vi "CRYReplace Stimulus Curve Name.vi"(7 "Setup in":T1={"No.VI"=0, "Category"="", "StepName"="", "Seq setup flattened"="", "Comment"="", "Steps config."=[], "Jump config"=[], "Start"=0.0, "Increment"=0.0, "Name"="Pa", "Unit"="Pa", "Y data"=1, "Y prefix"="", "Y dB ref"=1.0, "Y unit"="", "Repeat State Array"=[]} {"Repeat State Array"."Start" format="%#_5g"; "Y dB ref" format="%.1f"; "Y data" items=["dB", "Lin"]; "Start" format="%#_5g"}, 8 "Hardware Setup In":string, 9 "Step Setup In":string, 11 "Type In":string) -> (3 "Inserted Names Out":string[](array[string]))   [LabVIEW 2013]
uses:
  Typedef Control/CRYData Variant Array.ctl
  Typedef Control/CRYWaveform Cluster.ctl
  Typedef Control/CRYStep.ctl
  Typedef Control/CRYData Cluster.ctl
panel:
  in  "Wave out":T2[](array[typedef]) {"Y dB ref" format="%.1f"; "Y axis" items=["Log", "Lin"]; "Y data" items=["dB", "Lin"]; "X data" items=["dB", "Lin"]}
  in  "Data In":T3
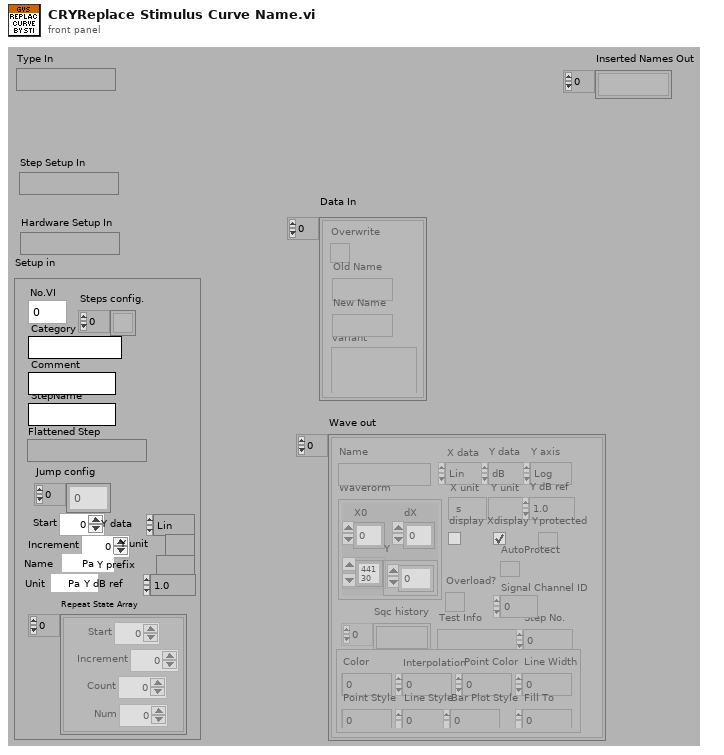
[diagram p1: front panel]
types:
  T1 = typedef "CRYStep.ctl" = cluster{"No.VI":i32, "Category":string, "StepName":string, "Seq setup flattened":string, "Comment":string, "Steps config.":bool[], "Jump config":i32[], "Start":dbl, "Increment":dbl, "Name":string, "Unit":string, "Y data":u16, "Y prefix":string, "Y dB ref":dbl, "Y unit":string, "Repeat State Array":cluster{"Start":dbl, "Increment":dbl, "Count":i32, "Num":i32}[]}
  T2 = typedef "CRYWaveform Cluster.ctl" = cluster{"Waveform":cluster{"X0":dbl, "dX":dbl, "Y":sgl[]}, "X data":u16, "Y data":u16, "Y axis":u16, "X unit":string, "Y unit":string, "Y dB ref":dbl, "display Y":bool, "display X":bool, "Overload?":bool, "Test Info":string, "Step No.":i32, "Name":string, "protected":bool, "Sqc history":string[], "Signal Channel ID":i32, "Plot Settings":cluster{"Color":u32, "Interpolation":u8, "Point Style":u8, "Line Style":u8, "Point Color":u32, "Line Width":u8, "Bar Plot Style":u8, "Fill To":i16}, "AutoProtect":bool}
  T3 = typedef "CRYData Variant Array.ctl" = cluster{"variant":variant, "Overwrite":bool, "Old Name":string, "New Name":string}[]
  T4 = typedef "CRYData Cluster.ctl" = cluster{"Name":string, "Curve":cluster{"x":dbl, "y":dbl, "z":dbl}[], "X data":u16, "Y data":u16, "Z data":u16, "X axis":u16, "Y axis":u16, "Z axis":u16, "X unit":string, "Y unit":string, "Z unit":string, "X dB ref":dbl, "Y dB ref":dbl, "Z dB ref":dbl, "single val":bool, "protected":bool, "display X":bool, "display Y":bool, "display Z":bool, "Test Info":string, "Step No.":i32, "Plot Settings":cluster{"Color":u32, "Interpolation":u8, "Point Style":u8, "Line Style":u8, "Point Color":u32, "Line Width":u8, "Bar Plot Style":u8, "Fill To":i16}, "AutoProtect":bool}
  T5 = cluster{"Start":dbl, "Increment":dbl, "Count":i32, "Num":i32}[]
  T6 = typedef "CRYStimulus Cluster.ctl" = cluster{"StimulusType":string, "UseMLValArray":u16[], "ML_axisArray":u16[], "MLValLevelNameArray":string[], "Level(U)Array":dbl[], "Start(Stop)FreqArray":dbl[], "Start(Stop)AmpArray":dbl[], "StepResolutionArray":u16[], "Unit_Array":u16[], "DegValArray":dbl[], "DegUnitArray":string[], "Steps1":i32, "Cycle/step1(#)":u32, "Time/step1(s)":dbl, "Transition1":dbl, "SweepRate2":dbl, "Freq3(Hz)":dbl, "Steps3(#)":dbl, "Cycles3(#)":u32, "StepSize3":dbl, "wave time":string, "RMS_Value4":dbl, "Peak_Value4":dbl, "WavePath4":string, "RMS_unit4":string, "Peak_unit4":string, "wave Info":string, "dc_ctrl5_1":u16, "dc_ctrl5_2":u16, "dc_polar5":u16, "Max.Current":u16, "Steps5(#)":u32, "Time/Step5":dbl, "Level5":dbl, "StepsSize5Val":dbl, "StepSize5Unit":string, "SweepType":u16, "Fixed/Ratio6":u16, "Transition6":dbl, "Steps6(#)":dbl, "Cycle/Steps6(#)":u32, "Time/Steps6(s)":dbl, "Freq6(Hz)":dbl, "Difference6(Hz)":dbl, "Ratio6":string, "NoiseType7":u16, "Duration7(s)":dbl, "MinFreq7(Hz)":dbl, "MaxFreq7(Hz)":dbl, "MinFreq8(Hz)":dbl, "MaxFreq8(Hz)":dbl, "FreqRounding8":bool, "Duration8(s)":dbl, "Tones8":dbl, "RoundingVal8":dbl, "ApplyEQ":bool, "Duration(s)":dbl, "CustomStimulusName ":string, "Flatten Element Array":string[], "sine waves":cluster{"freq":dbl, "ampl":dbl, "cycles":dbl}[], "Channel Out":i32, "RatioVal6":dbl, "TabCtrl6":enum32{"Master Tone", "Slave Tone"}, "Signal Type Name":string, "Help":string, "Channel Sel":u16, "V on DUT":bool, "Output Imp":dbl, "Nominal Imp":dbl}
  T7 = typedef "CRYStimulus Test Infor Cluster.ctl" = cluster{"Stimulus Type":string, "Signal Type":string, "In/Out":bool, "FAPS":cluster{"freq":dbl, "ampl":dbl, "cycles":dbl, "samples":i32}[], "Sampling Rate":dbl, "Samples":i32, "Analysis Param":string, "Resolution":u16, "Steps":u32, "Analysis Value":dbl[], "Diff Freq":dbl, "FStart":dbl, "FStop":dbl, "Calibration Param":string, "Anti Alias":dbl, "Level Out1":dbl, "Level Out2":dbl, "EQ":bool}
  T8 = typedef "CRYData Cluster Array.ctl" = T4[]
  T9 = typedef "CRYWaveform Cluster Array.ctl" = T2[]
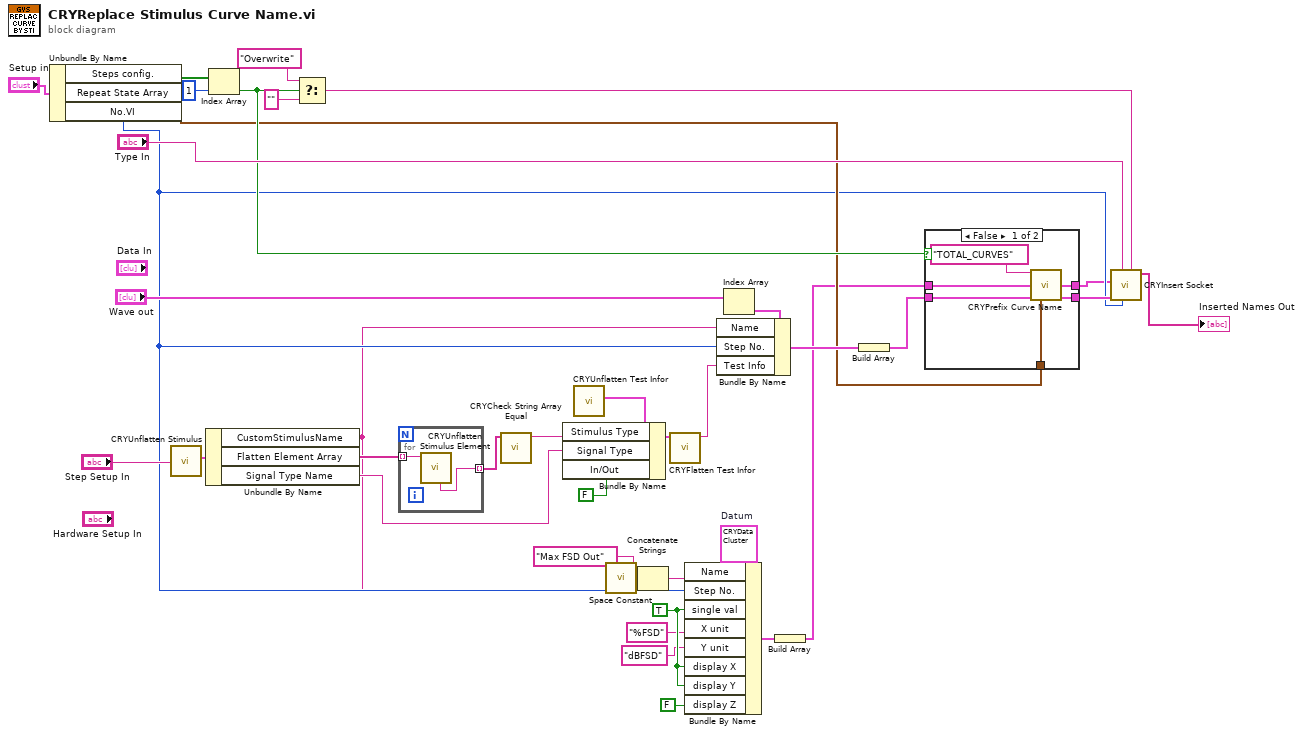
[diagram p0: block diagram]
diagram:
  w7 = T4 {"Name"="", "Curve"=[], "X data"=1, "Y data"=1, "Z data"=1, "X axis"=0, "Y axis"=1, "Z axis"=1, "X unit"="Hz", "Y unit"="", "Z unit"="deg.", "X dB ref"=1.0, "Y dB ref"=1.0, "Z dB ref"=1.0, "single val"=FALSE, "protected"=FALSE, "display X"=TRUE, "display Y"=TRUE, "display Z"=FALSE, "Test Info"="", "Step No."=0, "Plot Settings"={"Color"=0, "Interpolation"=0, "Point Style"=0, "Line Style"=0, "Point Color"=0, "Line Width"=0, "Bar Plot Style"=0, "Fill To"=0}, "AutoProtect"=FALSE}  # Datum
  w13 = TRUE ("single val")
  n1 = Unbundle By Name("Setup in") -> ("Steps config."=w18:bool[], "Repeat State Array"=w14:T5, "No.VI"=w5:i32)
  n2 = call "CRYUnflatten Stimulus.vi"("Flatten Stimulus"="Step Setup In") -> ("Stimulus"=w35:T6)  [unwired: 10 out]
  n3 = Unbundle By Name(w35) -> ("CustomStimulusName"=w4:string, "Flatten Element Array"=w34:string[], "Signal Type Name"=w28:string)
  n4 = Index Array(array=w18, index=1) -> (element=w15:bool)
  n5 = Select(t="Overwrite" ("Y unit"), s=w15, f="") -> (s? t:f=w20:string)
  n6 = for {
    tunnel: w34 -> [w40] mode=indexing
    tunnel: [w39] -> w33 mode=indexing
    n7 = call "CRYUnflatten Stimulus Element.vi"("Unflatten Stimulus Element setup"=w40) -> ("Type Name"=w39:string)  [unwired: 1 in, 9 out]
  }
  n8 = call "CRYCheck String Array Equal.vi"("In Array"=w33) -> ("Name String"=w32:string)  [unwired: 10 out]
  n9 = call "CRYUnflatten Test Infor.vi"() -> ("unflattened test infor data"=w31:T7)  [unwired: 1 in, 9 out]
  n10 = Bundle By Name(cluster=w31, "Stimulus Type"=w32, "Signal Type"=w28, "In/Out"=FALSE) -> (w30:T7)
  n11 = call <vilib>:"Space Constant.vi"() -> ("String"=w11:string)
  n12 = Concatenate Strings("Max FSD Out" ("Name"), w11, w4) -> (w6:string)
  n13 = call "CRYFlatten Test Infor.vi"("Test Infor data"=w30) -> ("Fattened Data"=w29:string)  [unwired: 10 out]
  n14 = Bundle By Name(cluster=w7, "Name"=w6, "Step No."=w5, "single val"=w13, "X unit"="%FSD", "Y unit"="dBFSD", "display X"=w13, "display Y"=w13, "display Z"=FALSE) -> (w3:T4)
  n15 = Index Array(array="Wave out") -> (element=w38:T2)  [unwired: 1 in]
  n16 = Bundle By Name(cluster=w38, "Name"=w4, "Step No."=w5, "Test Info"=w29) -> (w24:T2)
  n17 = Build Array(w3) -> (w2:T4[])
  n18 = Build Array(w24) -> (w17:T2[])
  n19 = case shown="False" w15 {
    tunnel: w17 -> [w45 w48]
    tunnel: [w44 w48] -> w16
    tunnel: w14 -> [w43 _]
    tunnel: w2 -> [w42 w47]
    tunnel: [w41 w47] -> w1
    frame False {
      n20 = call "CRYPrefix Curve Name.vi"("Type In"="TOTAL_CURVES", "Values In"=w42, "Waves In"=w45, "Repeat State Array In"=w43) -> ("Values Out"=w41:T8, "Waves Out"=w44:T9)  [unwired: 8 in, 2 out]
    }
    frame True {
    }
  }
  n21 = call "CRYInsert Socket.vi"("sOption2"=w20, "Step No."=w5, "sOption1"="Type In", "Waves"=w16, "Values"=w1) -> ("Inserted Names Out"=→"Inserted Names Out":string[])  [unwired: 6 in]
